vi "Test register value changed event.vi"(11 "Test Case In":refnum<class "Test Cases.lvclass">) -> (0 "error out":errorcluster, 3 "Test Case Out":refnum<class "Test Cases.lvclass">)   [LabVIEW 2024, in "Test Cases.lvclass"]
uses:
  Test Cases.lvclass
  Test Cases.lvclass/Test Cases.ctl
  source/Grid/SourceGrid.lvclass
  <vilib>/Astemes/LUnit/Test Case.lvclass
  source/Cells/Cell/Cell.lvclass
  source/Views/Cell View/Cell View.lvclass
  source/System.Drawing.Color.ctl
  source/SourceGrid.lvlib
  source/Editors/Combo Box/Combo Box.lvclass
  MyEventGrid/MyEventGrid.lvclass
  D:/git/Sourcegrid-LabVIEW/source/Grid/SourceGrid.lvclass
  D:/git/Sourcegrid-LabVIEW/tests/MyEventGrid/MyEventGrid.lvclass
  D:/git/Sourcegrid-LabVIEW/source/Editors/Editor Base/Editor Control Base.lvclass
  D:/git/Sourcegrid-LabVIEW/source/Editors/Combo Box/Combo Box.lvclass
  C:/Program Files/National Instruments/LabVIEW 2024/vi.lib/Astemes/LUnit/Test Case.lvclass
  C:/Program Files/National Instruments/LabVIEW 2024/vi.lib/Astemes/LUnit/LUnit Runnable.lvclass
  D:/git/Sourcegrid-LabVIEW/tests/Tests/Test Cases.lvclass
  D:/git/Sourcegrid-LabVIEW/dll/SourceGrid.dll
  dll/SourceGrid.dll
panel:
  in  "stop":bool
  in  "Grid Container":refnum<k24>(container)
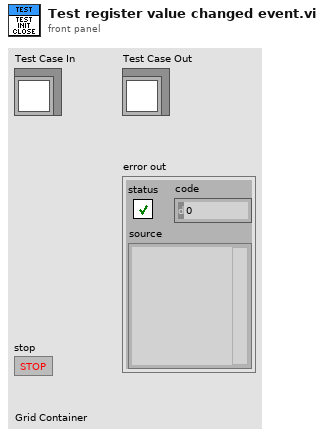
[diagram p1: front panel]
types:
  T1 = typedef "SourceGrid.lvlib/System.Drawing.Color.ctl" = enum16{"AliceBlue", "AntiqueWhite", "Aqua", "Aquamarine", "Azure", "Beige", "Bisque", "Black", "BlanchedAlmond", "Blue", "BlueViolet", "Brown", "BurlyWood", "CadetBlue", "Chartreuse", "Chocolate", "Coral", "CornflowerBlue", "Cornsilk", "Crimson", "Cyan", "DarkBlue", "DarkCyan", "DarkGoldenrod", "DarkGray", "DarkGreen", "DarkKhaki", "DarkMagenta", "DarkOliveGreen", "DarkOrange", "DarkOrchid", "DarkRed", "DarkSalmon", "DarkSeaGreen", "DarkSlateBlue", "DarkSlateGray", "DarkTurquoise", "DarkViolet", "DeepPink", "DeepSkyBlue", "DimGray", "DodgerBlue", "Firebrick", "FloralWhite", "ForestGreen", "Fuchsia", "Gainsboro", "GhostWhite", "Gold", "Goldenrod", "Gray", "Green", "GreenYellow", "Honeydew", "HotPink", "IndianRed", "Indigo", "Ivory", "Khaki", "Lavender", "LavenderBlush", "LawnGreen", "LemonChiffon", "LightBlue", "LightCoral", "LightCyan", "LightGoldenrodYellow", "LightGray", "LightGreen", "LightPink", "LightSalmon", "LightSeaGreen", "LightSkyBlue", "LightSlateGray", "LightSteelBlue", "LightYellow", "Lime", "LimeGreen", "Linen", "Magenta", "Maroon", "MediumAquamarine", "MediumBlue", "MediumOrchid", "MediumPurple", "MediumSeaGreen", "MediumSlateBlue", "MediumSpringGreen", "MediumTurquoise", "MediumVioletRed", "MidnightBlue", "MintCream", "MistyRose", "Moccasin", "NavajoWhite", "Navy", "OldLace", "Olive", "OliveDrab", "Orange", "OrangeRed", "Orchid", "PaleGoldenrod", "PaleGreen", "PaleTurquoise", "PaleVioletRed", "PapayaWhip", "PeachPuff", "Peru", "Pink", "Plum", "PowderBlue", "Purple", "Red", "RosyBrown", "RoyalBlue", "SaddleBrown", "Salmon", "SandyBrown", "SeaGreen", "SeaShell", "Sienna", "Silver", "SkyBlue", "SlateBlue", "SlateGray", "Snow", "SpringGreen", "SteelBlue", "Tan", "Teal", "Thistle", "Tomato", "Transparent", "Turquoise", "Violet", "Wheat", "White", "WhiteSmoke", "Yellow"}
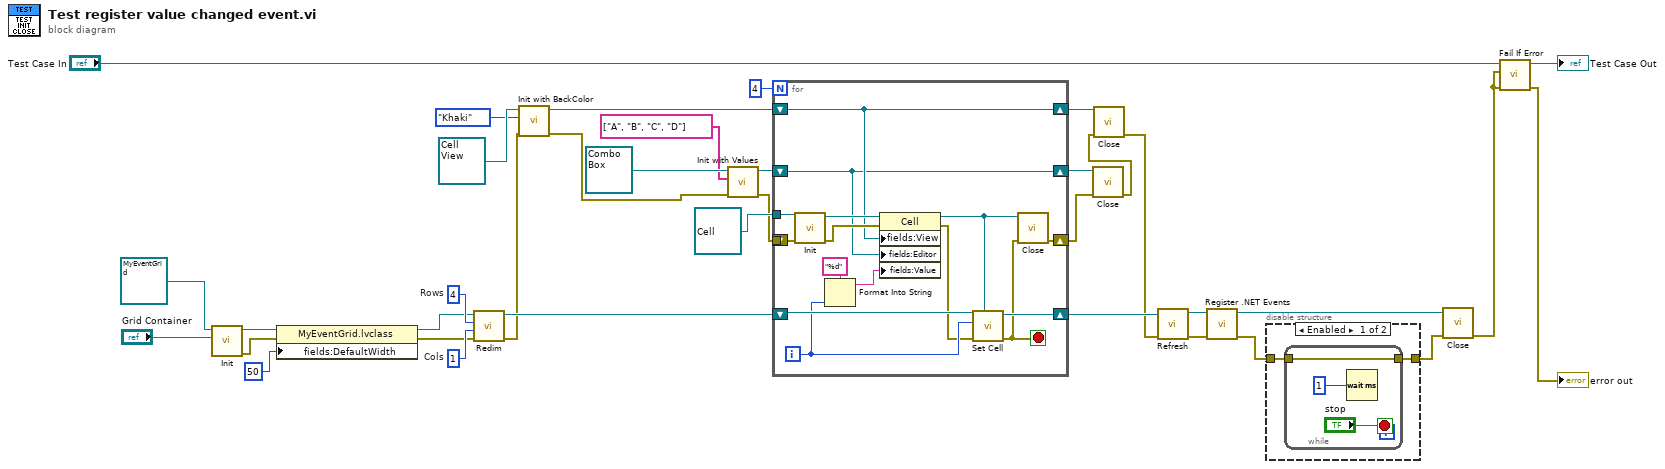
[diagram p0: block diagram]
diagram:
  w32 = 1  # Cols
  w33 = 4  # Rows
  n1 = call-dynamic "Init.vi"("Sourcegrid Container"="Grid Container", "Grid in"=refnum<class "MyEventGrid.lvclass"> refnum) -> ("error out"=w21:errorcluster, "Grid out"=w29:refnum<class "MyEventGrid.lvclass">)  [unwired: 8 in]
  n2 = property class="MyEventGrid.lvclass"(reference=w29, error in=w21, "fields:DefaultWidth"=50 ("DefaultWidth")) -> (reference out=w28:refnum<class "MyEventGrid.lvclass">, error out=w27:errorcluster)
  n3 = call "Redim.vi"("error in"=w27, "Columns"=w32, "Rows"=w33, "Sourcegrid in"=w28) -> ("error out"=w9:errorcluster, "Sourcegrid out"=w24:refnum<class "MyEventGrid.lvclass">)  [unwired: 6 in]
  n4 = call-dynamic "Init with BackColor.vi"("error in"=w9, "Color"=System.Drawing.Color."Khaki", "Cell View in"=refnum<class "Cell View.lvclass"> refnum) -> ("error out"=w17:errorcluster, "Cell View out"=w11:refnum<class "Cell View.lvclass">)  [unwired: 7 in]
  n5 = call-dynamic "Init with Values.vi"("error in"=w17, "Values"=string[] ["A", "B", "C", "D"], "Combo Box in"=refnum<class "Combo Box.lvclass"> refnum ("SourceGrid.lvlib:Combo Box.lvclass")) -> ("error out"=w12:errorcluster, "Combo Box out"=w14:refnum<class "Combo Box.lvclass">)  [unwired: 7 in]
  n6 = for {
    N: 4 -> [_]
    shift-right: [w49] -> w7
    shift-left: _ -> [_]
    shift-right: [w51] -> w25
    shift-left: w24 -> [w50]
    tunnel: refnum<class "Cell.lvclass"> refnum ("Cell in") -> [w44]
    tunnel: w12 -> [w46]
    shift-right: [w39] -> w10
    shift-left: w11 -> [w39]
    shift-right: [w38] -> w8
    shift-left: w14 -> [w38]
    i -> [w47]
    stop <- w37 stop-if-true
    n7 = call-dynamic "Init.vi"("error in"=w46, "Cell in"=w44) -> ("error out"=w41:errorcluster, "Cell out"=w43:refnum<class "Cell.lvclass">)  [unwired: 8 in]
    n8 = Format Into String(format string="%d", w47) -> (resulting string=w40:string)  [unwired: 2 in, 1 out]
    n9 = property class="Cell"(reference=w43, error in=w41, "fields:View"=w39, "fields:Editor"=w38, "fields:Value"=w40) -> (reference out=w42:refnum<class "Cell.lvclass">, error out=w45:errorcluster)
    n10 = call "Set Cell.vi"("Cell"=w42, "error in"=w45, "Row"=w47, "Sourcegrid in"=w50) -> ("error out"=w37:errorcluster, "Sourcegrid out"=w51:refnum<class "MyEventGrid.lvclass">)  [unwired: 6 in]
    n11 = call-dynamic "Close.vi"("error in"=w37, "Cell in"=w42) -> ("error out"=w49:errorcluster)  [unwired: 8 in, 1 out]
  }
  n12 = call-dynamic "Close.vi"("error in"=w7, "Combo Box in"=w8) -> ("error out"=w6:errorcluster)  [unwired: 8 in, 1 out]
  n13 = call-dynamic "Close.vi"("error in"=w6, "Cell View in"=w10) -> ("error out"=w16:errorcluster)  [unwired: 8 in, 1 out]
  n14 = call "Refresh.vi"("error in"=w16, "SourceGrid in"=w25) -> ("error out"=w5:errorcluster, "SourceGrid out"=w2:refnum<class "MyEventGrid.lvclass">)  [unwired: 8 in]
  n15 = call-dynamic "Register .NET Events.vi"("error in"=w5, "MyEventGrid in"=w2) -> ("error out"=w3:errorcluster, "MyEventGrid out"=w1:refnum<class "MyEventGrid.lvclass">)  [unwired: 8 in]
  n16 = disable-structure shown="Enabled" {
    disable-tunnel: w3 -> [w53 w57]
    disable-tunnel: [w52 w57] -> w4
    frame Enabled {
      n17 = while {
        tunnel: w53 -> [w54]
        tunnel: [w54] -> w52
        stop <- "stop" stop-if-true
        n18 = Wait (ms)(milliseconds to wait=u32 1) -> ()  [unwired: 1 out]
      }
    }
    frame Disabled {
    }
  }
  n19 = call-dynamic "Close.vi"("error in"=w4, "Sourcegrid in"=w1) -> ("error out"=w31:errorcluster)  [unwired: 8 in, 1 out]
  n20 = call <vilib>:"Fail If Error.vi"("error in (no error)"=w31, "Assert error"=w31, "LUnit Test Case In"="Test Case In") -> ("error out"=→"error out":errorcluster, "LUnit Test Case Out"=→"Test Case Out":refnum<class "Test Cases.lvclass">)  [unwired: 7 in]
